vi "Do.vi"(0 "ControlDoBase in":refnum<class "ControlActionBase.lvclass">, 5 "VI Reference in":refnum<vi>, 7 "Control Path":string[](array[string]), 11 "error in":errorcluster) -> (4 "ControlDoBase out":refnum<class "ControlActionBase.lvclass">, 6 "VI Reference out":refnum<vi>, 15 "error out":errorcluster)   [LabVIEW 2016, in "ControlActionBase.lvclass"]
doc: "This VI sets the value of controls present in the other VI . It is mainly used to set values of controls present inside tabs and clusters."
uses:
  ControlActionBase.lvclass
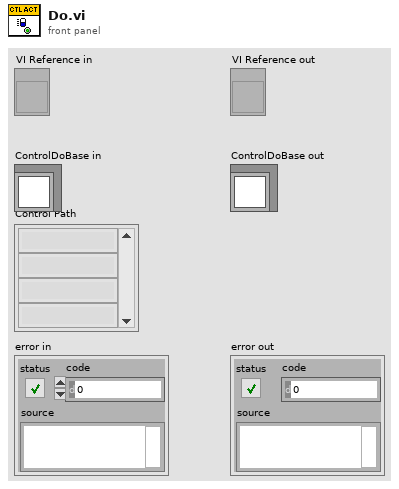
[diagram p1: front panel]
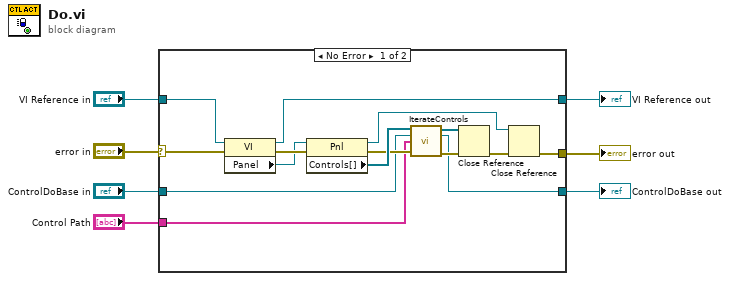
[diagram p0: block diagram]
diagram:
  n1 = case shown="No Error" "error in" {
    selector: "error in" -> [w20 w25]
    tunnel: [w19 w24] -> w6
    tunnel: [w18 w25] -> w5
    tunnel: "VI Reference in" -> [w16 w24]
    tunnel: "Control Path" -> [w8 _]
    tunnel: "ControlDoBase in" -> [w10 w23]
    tunnel: [w9 w23] -> w1
    frame No Error {
      n2 = property class="VI"(reference=w16, error in=w20) -> (reference out=w19:refnum<vi>, error out=w22:errorcluster, "Panel"=w21:refnum<vi>)
      n3 = property class="Pnl"(reference=w21, error in=w22) -> (reference out=w17:refnum<vi>, error out=w14:errorcluster, "Controls[]"=w15:refnum<vi>[])
      n4 = call-dynamic "IterateControls.vi"("Controls[] In"=w15, "ControlDoBase in"=w10, "Control Path"=w8, "error in (no error)"=w14) -> ("Controls[] Out"=w11:refnum<vi>[], "ControlDoBase out"=w9:refnum<class "ControlActionBase.lvclass">, "error out"=w13:errorcluster)  [unwired: 9 in]
      n5 = Close Reference(reference=w11, error in (no error)=w13) -> (error out=w12:errorcluster)
      n6 = Close Reference(reference=w17, error in (no error)=w12) -> (error out=w18:errorcluster)
    }
    frame Error {
    }
  }
  "VI Reference out" <- w6
  "error out" <- w5
  "ControlDoBase out" <- w1
